vi "locl_variable_test.vi"() -> ()   [LabVIEW 2014]
panel:
  out "data out":dbl[](array[numeric])
  in  "stop":bool
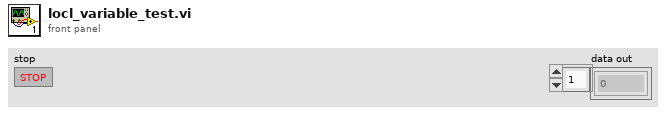
[diagram p1: front panel]
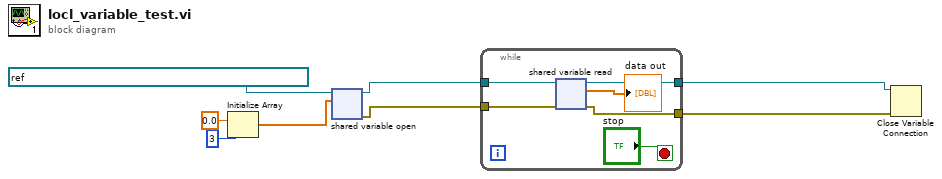
[diagram p0: block diagram]
diagram:
  n1 = Initialize Array(0.0 ("element"), 3 ("dimension size")) -> (w1:dbl[])
  n2 = shared-variable-open(refnum<k21> "ni.var.psp://localhost/synth_settings/synth_settings" ("shared variable refnum in"), w1) -> (w8:refnum<k21>, w5:errorcluster)  [unwired: 2 in]
  n3 = while {
    tunnel: w8 -> [w14]
    tunnel: [w13] -> w7
    tunnel: w5 -> [w12]
    tunnel: [w11] -> w4
    stop <- "stop" stop-if-true
    n4 = shared-variable-read(w14, w12) -> (w13:refnum<k21>, w11:errorcluster, →"data out":dbl[])  [unwired: 1 out]
  }
  n5 = Close Variable Connection(8:w4, 11:w7) -> ()  [unwired: 1 out]
